vi "VendingMachine.vi"() -> ()   [LabVIEW 2010]
panel:
  in  "Kabooom":bool
  out "Result":string
  in  "spend1Coin":bool
  out "coinsDropped":i32
  in  "dropCoinButton":bool
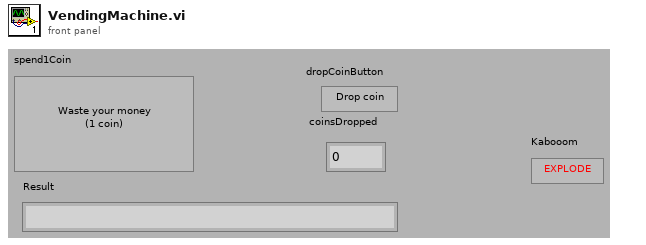
[diagram p1: front panel]
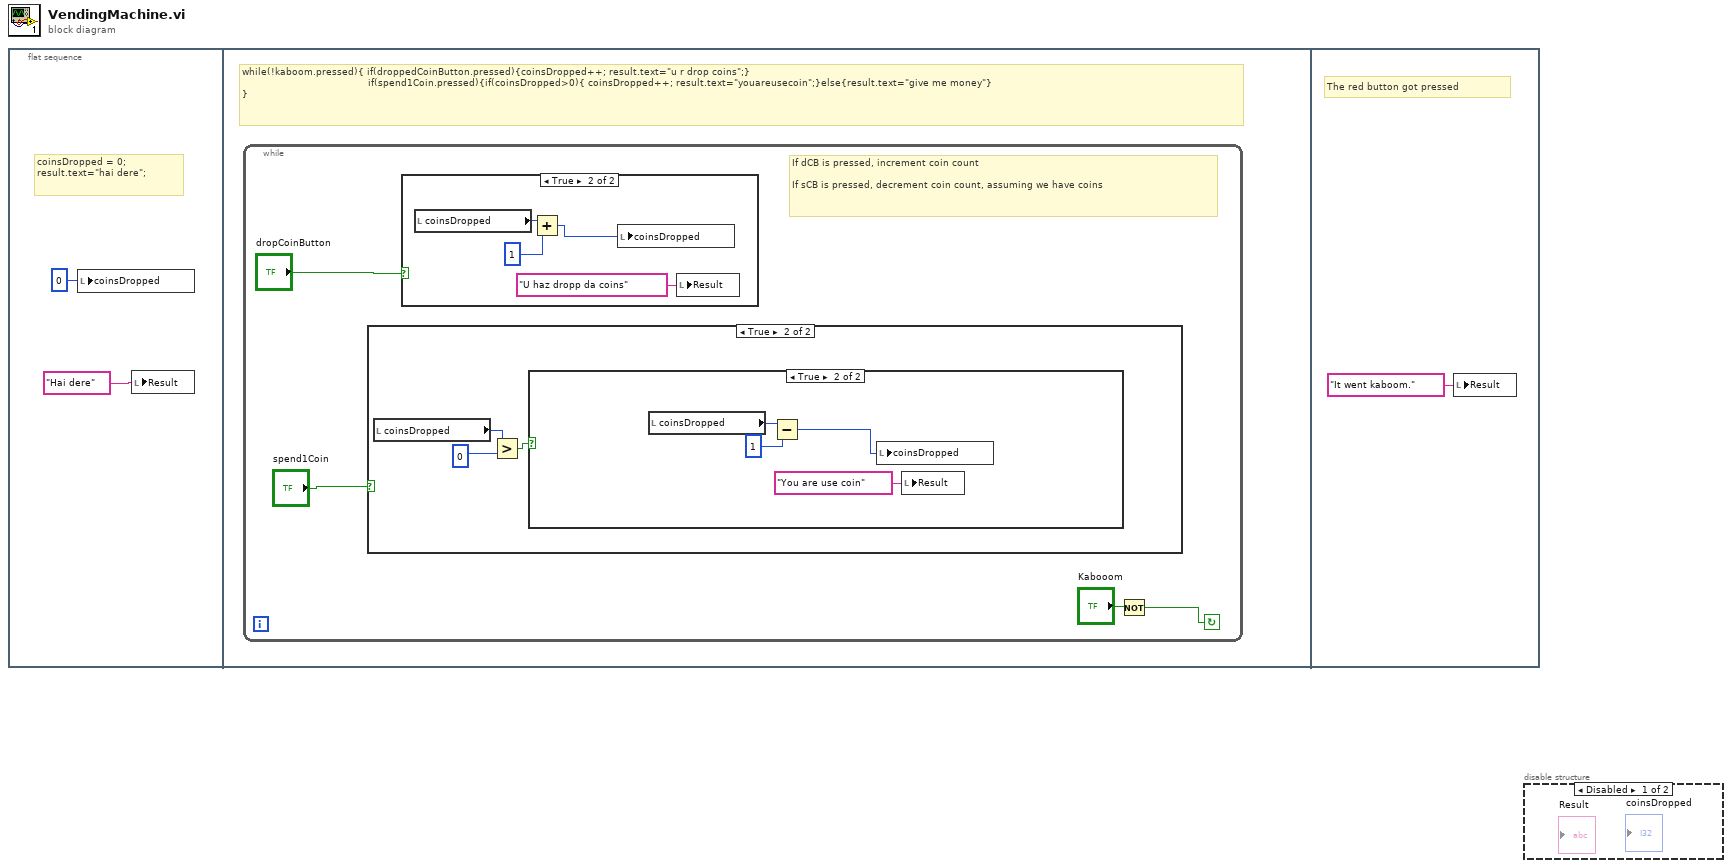
[diagram p0: block diagram]
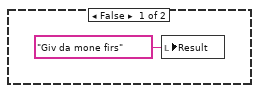
[diagram p4: hidden frame]
diagram:
  n1 = flat-sequence {
    frame #0 {
      # "coinsDropped = 0;\nresult.text=\"hai dere\";"
      n2 = local write "coinsDropped"(0 ("coinsDropped")) -> ()
      n3 = local write "Result"("Hai dere" ("Result")) -> ()
    }
    frame #1 {
      # "while(!kaboom.pressed){ if(droppedCoinButton.pressed){coinsDropped++; result.text=\"u r drop coins\";} \n                                          if(spend1Coin.pressed){if(coinsDropped>0){ coinsDropped++; result.text=\"youareusecoin\";}else{result.text=\"give me money\"}\n}"
      n4 = while {
        stop <- w3 continue-if-true
        # "If dCB is pressed, increment coin count\n\nIf sCB is pressed, decrement coin count, assuming we have coins"
        n5 = case shown="True" "spend1Coin" {
          frame False {
          }
          frame True {
            n6 = local read "coinsDropped"() -> (w9:i32)
            n7 = Greater?(x=w9, y=0) -> (0:w7:bool)
            n8 = case shown="True" w7 {
              frame False {
                n9 = local write "Result"("Giv da mone firs" ("Result")) -> ()
              }
              frame True {
                n10 = local read "coinsDropped"() -> (w14:i32)
                n11 = Subtract(x=w14, y=1) -> (x-y=w12:i32)
                n12 = local write "coinsDropped"(w12) -> ()
                n13 = local write "Result"("You are use coin" ("Result")) -> ()
              }
            }
          }
        }
        n14 = case shown="True" "dropCoinButton" {
          frame False {
          }
          frame True {
            n15 = local read "coinsDropped"() -> (w18:i32)
            n16 = Add(x=w18, y=1) -> (x+y=w16:i32)
            n17 = local write "coinsDropped"(w16) -> ()
            n18 = local write "Result"("U haz dropp da coins" ("Result")) -> ()
          }
        }
        n19 = Not(x="Kabooom") -> (.not. x?=w3:bool)
      }
    }
    frame #2 {
      # "The red button got pressed"
      n20 = local write "Result"("It went kaboom." ("Result")) -> ()
    }
  }
  n21 = disable-structure shown="Disabled" {
    frame Disabled {
    }
    frame Enabled {
    }
  }
